vi "Wait_s.vi"(7 "Time to wait":i32 caption="Time to wait [s]" min=0, 9 "Skip wait on error?":bool=TRUE caption="Skip wait on error? (T)", 11 "Error in":errorcluster caption="Error in (no error)", 12 "Skip wait?":bool caption="Skip wait? (F)", 13 "Abort wait on occurrence":refnum<k4> caption="Abort wait on occurrence (none)") -> (15 "Error out":errorcluster)   [LabVIEW 2017, in "GPTiming.lvlib"]
doc: "Waits <B>Time to wait</B>. Select a polymorphic instance of either hours, minutes, seconds, milliseconds, milliseconds (Real-Time) or microseconds (Real-Time) by right-clicking the function.\n\nIf you wire an occurrence to the optional <B>Abort wait on occurrence</B> input you can abort the wait prematurely by setting that occurrence.\n\nThe effect of setting <B>Time to wait</B> to a negative value depends on if you have specified an abort occurrence or not. If an abort occurrence is specified a negative <B>Time to wait</B> will make this function wait indefinetely until abort is asserted. If an abort occurrence is not specified a negative <B>Time to wait</B> will be coerced to zero making this function end immediately. This setup is chosen to protect from setting a timeout value that you can't get out of.\n\nThis VI is inlined. It skips the wait if there is an error on <B>Error in</B> AND <B>Skip wait on error?</B> is True (which is the default). It also skips the wait unconditionally if <B>Skip wait?</B> is True.\n\n<B>Note</B>\nThe non-Real-Time version (which works both on Desktop and on Real-Time) of this function yields control of the execution thread during the wait, but it behaves differently on Windows and on Real-Time. On Windows, the function waits up to the value specified in <B>Time to wait</B>. On Real-Time the function waits at least the value specified in <B>Time to wait</B>. This function has a margin of error of plus or minus one millisecond.\n\n<B>Note</B> (Real-Time)\nThe Real-Time versions of this function blocks the execution of the thread of the calling VI. Any code running in parallel in the calling VI or any VIs running in the same execution system thread are unable to execute during the time that these functions wait.\n\nSteen Schmidt\nGPower\n2/11 2014"
uses:
  GPTiming.lvlib
  Error/GPError.lvlib
panel:
  # "Copyright © 2014\nGPower\nSee enclosed license file for terms and conditions"
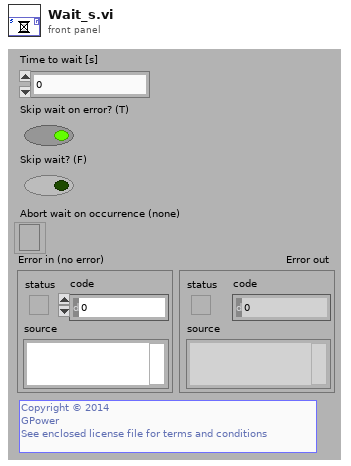
[diagram p1: front panel]
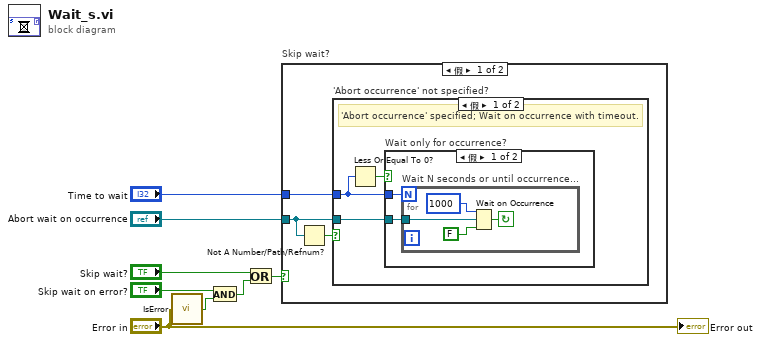
[diagram p0: block diagram]
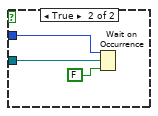
[diagram p2: hidden frame]
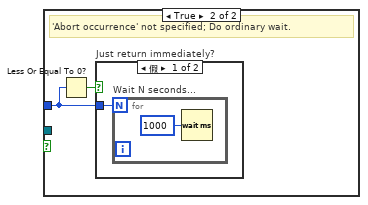
[diagram p3: hidden frame]
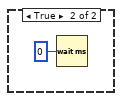
[diagram p4: hidden frame]
diagram:
  n1 = call "IsError.vi"("Error in"="Error in") -> ("Error?"=w6:bool)  [unwired: 4 in]
  n2 = And(x="Skip wait on error?", y=w6) -> (x .and. y?=w4:bool)
  n3 = Or(x="Skip wait?", y=w4) -> (x .or. y?=w3:bool)
  n4 = case "Skip wait?" shown="假" w3 {
    tunnel: "Time to wait" -> [w9 _]
    tunnel: "Abort wait on occurrence" -> [w10 _]
    frame False {
      n5 = Not A Number/Path/Refnum?(number/path/refnum=w10) -> (NaN/Path/Refnum?=w11:bool)
      n6 = case "'Abort occurrence' not specified?" shown="假" w11 {
        tunnel: w9 -> [w13 w24]
        tunnel: w10 -> [w12 _]
        frame False {
          # "'Abort occurrence' specified; Wait on occurrence with timeout."
          n7 = Less Or Equal To 0?(x=w13) -> (x <= 0?=w14:bool)
          n8 = case "Wait only for occurrence?" shown="假" w14 {
            tunnel: w13 -> [w16 w21]
            tunnel: w12 -> [w15 w22]
            frame False {
              n9 = for "Wait N seconds or until occurrence..." {
                N: w16 -> [_]
                tunnel: w15 -> [w19]
                stop <- w17 continue-if-true
                n10 = Wait on Occurrence(1:FALSE ("ignore previous (T)"), 2:w19, 3:1000 ("milliseconds to wait")) -> (0:w17:bool)
              }
            }
            frame True {
              n11 = Wait on Occurrence(1:FALSE ("ignore previous (T)"), 2:w22, 3:w21) -> ()  [unwired: 1 out]
            }
          }
        }
        frame True {
          # "'Abort occurrence' not specified; Do ordinary wait."
          n12 = Less Or Equal To 0?(x=w24) -> (x <= 0?=w25:bool)
          n13 = case "Just return immediately?" shown="假" w25 {
            tunnel: w24 -> [w26 _]
            frame False {
              n14 = for "Wait N seconds..." {
                N: w26 -> [_]
                n15 = Wait (ms)(milliseconds to wait=u32 1000) -> ()  [unwired: 1 out]
              }
            }
            frame True {
              n16 = Wait (ms)(milliseconds to wait=u32 0) -> ()  [unwired: 1 out]
            }
          }
        }
      }
    }
    frame True {
    }
  }
  "Error out" <- "Error in"
